vi "Write Shunt Resistor Location.vi"(8 "error in (no error)":errorcluster, 10 "Shunt Resistor Location":i32(ring)=-1 items=["default"=-1, "Internal"=10200, "External"=10167], 11 "BNT_ULx-MCSV-I in":refnum<class "BNT_ULx-MCSV-I.lvclass">) -> (0 "error out":errorcluster, 3 "BNT_ULx-MCSV-I out":refnum<class "BNT_ULx-MCSV-I.lvclass">)   [LabVIEW 2020, in "BNT_ULx.lvlib" / "BNT_ULx-MCSV-I.lvclass"]
doc: "Write shunt resistor location."
uses:
  BNT_ULx-MCSV-I.lvclass
  BNT_ULx-MCSV-I.lvclass/BNT_ULx-MCSV-I.ctl
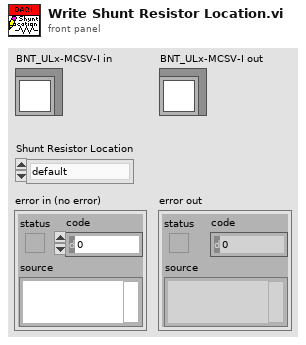
[diagram p1: front panel]
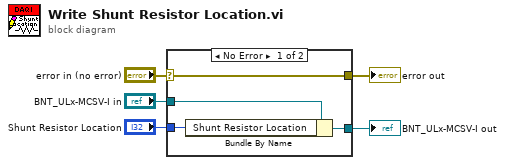
[diagram p0: block diagram]
diagram:
  n1 = case shown="No Error" "error in (no error)" {
    selector: "error in (no error)" -> [w9 w10]
    tunnel: [w9 w10] -> w4
    tunnel: [w7 w11] -> w2
    tunnel: "BNT_ULx-MCSV-I in" -> [w8 w11]
    tunnel: "Shunt Resistor Location" -> [w6 _]
    frame No Error {
      n2 = Bundle By Name(cluster=w8, "Shunt Resistor Location"=w6) -> (w7:refnum<class "BNT_ULx-MCSV-I.lvclass">)
    }
    frame Error {
    }
  }
  "error out" <- w4
  "BNT_ULx-MCSV-I out" <- w2
